vi "calculate.vi"(8 "error in (no error)":errorcluster, 10 "Data":u8[](array[numeric]), 11 "CRC in":refnum<class "CRC.lvclass">) -> (0 "error out":errorcluster, 2 "CRC":u16 format="%x", 3 "CRC out":refnum<class "CRC.lvclass">)   [LabVIEW 2016, in "CRC.lvclass"]
uses:
  CRC.lvclass
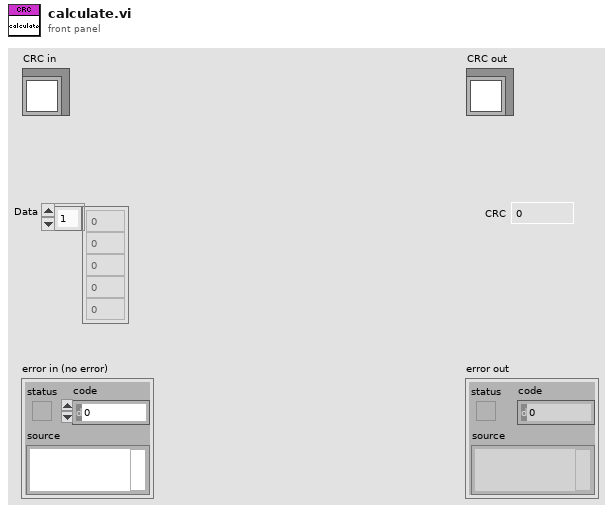
[diagram p1: front panel]
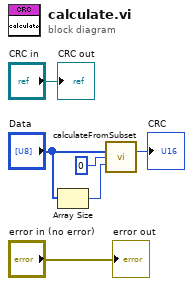
[diagram p0: block diagram]
diagram:
  n1 = Array Size(array="Data") -> (size(s)=w4:i32)
  n2 = call "calculateFromSubset.vi"("Data"="Data", "StartIndex"=0, "Length"=w4) -> ("CRC"=→"CRC":u16)  [unwired: 10 in, 2 out]
  "error out" <- "error in (no error)"
  "CRC out" <- "CRC in"
